vi "PH_PP_CurrentMeas.PC read RT Client 3.vi"(0 "i ref in":refnum<vi>, 5 "error in (no error)":errorcluster) -> (14 "i ref out":refnum<vi>, 16 "Data PA":waveform(dbl)[](array[waveform]), 17 "Data MA FR":waveform(dbl)[](array[waveform]), 18 "Data MA Ground":waveform(dbl)[](array[waveform]), 19 "error out":errorcluster)   [LabVIEW 2014, in "PH_PP_CurrentMeas.lvlib"]
doc: "This VI reads out the data of RT client 1."
uses:
  PH_PP_CurrentMeas.lvlib
panel:
  in  "Array":waveform(dbl)[](array[waveform])
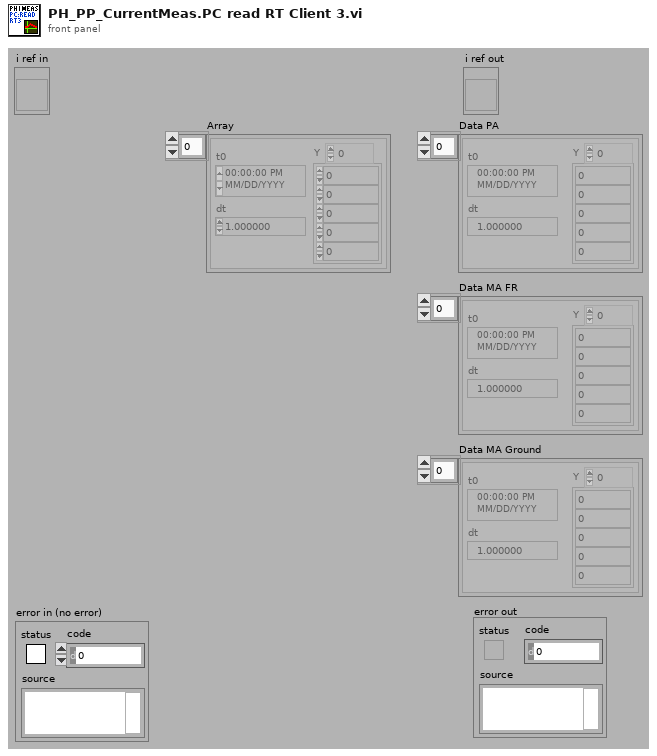
[diagram p1: front panel]
types:
  T1 = typedef "PH_PP_CurrentMeas.lvlib/PH_PP_CurrentMeas.i attribute.ctl" = cluster{"Status":cluster{"GUI Ref Hardware Feedback":refnum<vi>, "Tab Control":refnum<vi>}, "PU 1":cluster{"Instance":string, "Status":T2, "Ref Status ":refnum<vi>, "Data":waveform(dbl)[], "Ref Data":refnum<vi>}, "PU 2":cluster{"Instance":string, "Status":T2, "Ref Status ":refnum<vi>, "Data":waveform(dbl)[], "Ref Data":refnum<vi>}, "PU 3":cluster{"Instance":string, "Status":T2, "Ref Status ":refnum<vi>, "Data":waveform(dbl)[], "Ref Data":refnum<vi>}, "PU 4":cluster{"Instance":string, "Status":T2, "Ref Status ":refnum<vi>, "Data":waveform(dbl)[], "Ref Data":refnum<vi>}, "PU 5":cluster{"Instance":string, "Status":T2, "Ref Status ":refnum<vi>, "Data":waveform(dbl)[], "Ref Data":refnum<vi>}, "FR":cluster{"Instance":string, "Status":T2, "Ref Status ":refnum<vi>, "Data":waveform(dbl)[], "Ref Data":refnum<vi>}, "PA - 19mm 1":cluster{"Instance":string, "Status":T2, "Ref Status ":refnum<vi>}, "PA - 19mm 2":cluster{"Instance":string, "Status":T2, "Ref Status ":refnum<vi>, "no link":bool}, "PA - 45mm":cluster{"Instance":string, "Status":T2, "Ref Status ":refnum<vi>, "no link":bool}, "PA Data":cluster{"Data":waveform(dbl)[], "Ref":refnum<vi>}, "Sequencer":cluster{"Instance":string, "SM State Ref":refnum<vi>}, "Tasks":cluster{"Port":u16, "connection ID":refnum<k5>, "Status":T2, "Ref":refnum<vi>, "Ref Bar":refnum<vi>, "Feedback":cluster{"Received Data Sets":T3[], "Driver Error":errorcluster, "Connection not established":bool, "Error unpacking the data":bool, "No Task defined":bool, "Not triggered yet":bool}, "Data":waveform(dbl)[], "Ref Teststart Task":refnum<vi>}[], "in use":cluster{"MA DP":bool, "FR and PA":bool}, "DAQ Server":string}
  T2 = typedef "PH_StatusHandler.lvlib/PH_StatusHandler.Status.ctl" = i16
  T3 = typedef "PH_PP_CurrentMeas.lvlib/PH_PP_CurrentMeas.CommandCluster.ctl" = cluster{"Command":string, "Data":string, "error out":errorcluster}
  T4 = cluster{"Port":u16, "connection ID":refnum<k5>, "Status":T2, "Ref":refnum<vi>, "Ref Bar":refnum<vi>, "Feedback":cluster{"Received Data Sets":T3[], "Driver Error":errorcluster, "Connection not established":bool, "Error unpacking the data":bool, "No Task defined":bool, "Not triggered yet":bool}, "Data":waveform(dbl)[], "Ref Teststart Task":refnum<vi>}[]
  T5 = cluster{"Port":u16, "connection ID":refnum<k5>, "Status":T2, "Ref":refnum<vi>, "Ref Bar":refnum<vi>, "Feedback":cluster{"Received Data Sets":T3[], "Driver Error":errorcluster, "Connection not established":bool, "Error unpacking the data":bool, "No Task defined":bool, "Not triggered yet":bool}, "Data":waveform(dbl)[], "Ref Teststart Task":refnum<vi>}
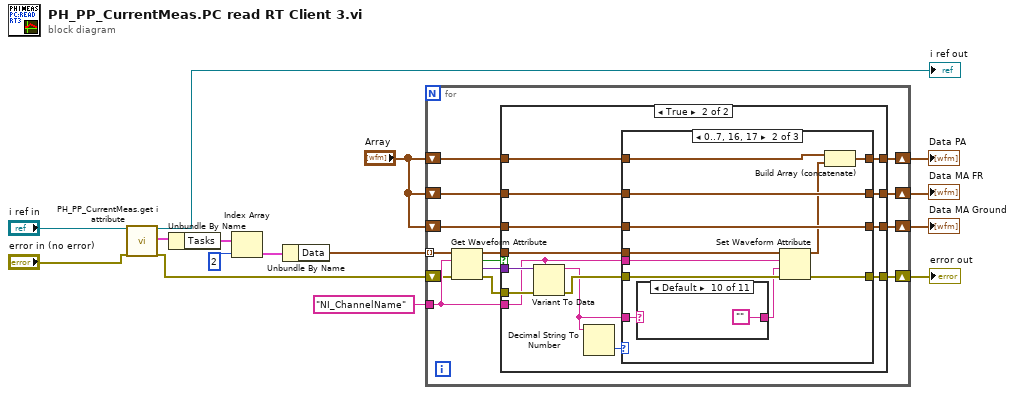
[diagram p0: block diagram]
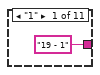
[diagram p4: hidden frame]
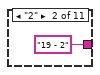
[diagram p5: hidden frame]
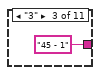
[diagram p6: hidden frame]
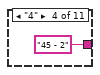
[diagram p7: hidden frame]
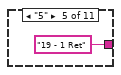
[diagram p8: hidden frame]
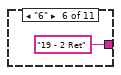
[diagram p9: hidden frame]
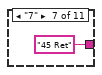
[diagram p10: hidden frame]
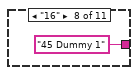
[diagram p11: hidden frame]
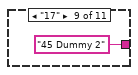
[diagram p12: hidden frame]
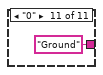
[diagram p13: hidden frame]
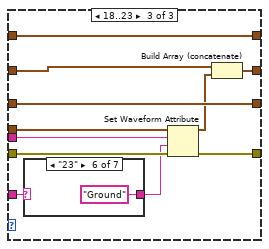
[diagram p14: hidden frame]
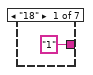
[diagram p15: hidden frame]
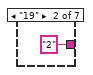
[diagram p16: hidden frame]
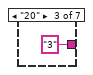
[diagram p17: hidden frame]
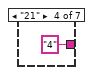
[diagram p18: hidden frame]
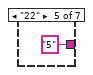
[diagram p19: hidden frame]
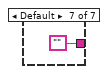
[diagram p20: hidden frame]
diagram:
  n1 = call "PH_PP_CurrentMeas.get i attribute.vi"("i ref in"="i ref in", "error in (no error)"="error in (no error)") -> ("i ref out"=→"i ref out":refnum<vi>, "i attribute"=w15:T1, "error out"=w3:errorcluster)  [unwired: 15 in]
  n2 = Unbundle By Name(w15) -> ("Tasks"=w12:T4)
  n3 = Index Array(array=w12, index=2) -> (element=w2:T5)
  n4 = Unbundle By Name(w2) -> ("Data"=w1:waveform(dbl)[])
  n5 = for {
    tunnel: w1 -> [w19] mode=indexing
    tunnel: "NI_ChannelName" ("name") -> [w22]
    shift-right: [w29] -> w10
    shift-left: w3 -> [w17]
    shift-right: [w28] -> w8
    shift-left: "Array" -> [w27]
    shift-right: [w26] -> w7
    shift-left: "Array" -> [w25]
    shift-right: [w24] -> w6
    shift-left: "Array" -> [w23]
    n6 = Get Waveform Attribute(4:w17, 6:w22, 7:w19) -> (0:w16:errorcluster, 1:w21:variant, 2:w20:bool, 3:w18:waveform(dbl))  [unwired: 1 in]
    n7 = case shown="True" w20 {
      tunnel: w18 -> [_ w47]
      tunnel: w16 -> [w33 w38]
      tunnel: [w33 w46] -> w29
      tunnel: w21 -> [_ w36]
      tunnel: w22 -> [_ w34]
      tunnel: [w32 w44] -> w28
      tunnel: w27 -> [w32 w43]
      tunnel: [w31 w42] -> w26
      tunnel: w25 -> [w31 w41]
      tunnel: [w30 w40] -> w24
      tunnel: w23 -> [w30 w39]
      frame False {
      }
      frame True {
        n8 = Variant To Data(error in=w38, type=w34, Variant=w36) -> (data=w35:string, error out=w37:errorcluster)
        n9 = Decimal String To Number(string=w35) -> (number=w45:i32)  [unwired: 2 in, 1 out]
        n10 = case shown="0..7, 16, 17" w45 {
          tunnel: w47 -> [_ w57 w79]
          tunnel: [w50 w55 w76] -> w46
          tunnel: w34 -> [_ w52 w74]
          tunnel: w37 -> [w50 w54 w77]
          tunnel: [w51 w62 w83] -> w44
          tunnel: w43 -> [w51 w61 w83]
          tunnel: w35 -> [_ w60 w84]
          tunnel: [w49 w59 w82] -> w42
          tunnel: w41 -> [w49 w59 w81]
          tunnel: [w48 w58 w80] -> w40
          tunnel: w39 -> [w48 w58 w80]
          frame Default {
          }
          frame 0..7, 16, 17 {
            n11 = case shown="Default" w60 {
              tunnel: ["19 - 1" "19 - 2" "45 - 1" "45 - 2" "19 - 1 Ret" "19 - 2 Ret" "45 Ret" "45 Dummy 1" "45 Dummy 2" "" "Ground"] -> w53
              frame "1" {
              }
              frame "2" {
              }
              frame "3" {
              }
              frame "4" {
              }
              frame "5" {
              }
              frame "6" {
              }
              frame "7" {
              }
              frame "16" {
              }
              frame "17" {
              }
              frame Default {
              }
              frame "0" {
              }
            }
            n12 = Set Waveform Attribute(4:w54, 5:w53, 6:w52, 7:w57) -> (0:w55:errorcluster, 3:w56:waveform(dbl))  [unwired: 1 out]
            n13 = Build Array (concatenate)(w61, w56) -> (w62:waveform(dbl)[])
          }
          frame 18..23 {
            n14 = case shown="\"23\"" w84 {
              tunnel: ["1" "2" "3" "4" "5" "Ground" ""] -> w75
              frame "18" {
              }
              frame "19" {
              }
              frame "20" {
              }
              frame "21" {
              }
              frame "22" {
              }
              frame "23" {
              }
              frame Default {
              }
            }
            n15 = Set Waveform Attribute(4:w77, 5:w75, 6:w74, 7:w79) -> (0:w76:errorcluster, 3:w78:waveform(dbl))  [unwired: 1 out]
            n16 = Build Array (concatenate)(w81, w78) -> (w82:waveform(dbl)[])
          }
        }
      }
    }
  }
  "error out" <- w10
  "Data PA" <- w8
  "Data MA FR" <- w7
  "Data MA Ground" <- w6
